vi "查找文件或文件夹.vi"(6 "create file or folder？":bool=TRUE, 8 "error in":errorcluster, 11 "pathIn":path caption="路径") -> (0 "error out":errorcluster, 2 "file or folder exists?":bool caption="文件或文件夹存在？", 3 "pathOut":path)   [LabVIEW 2014]
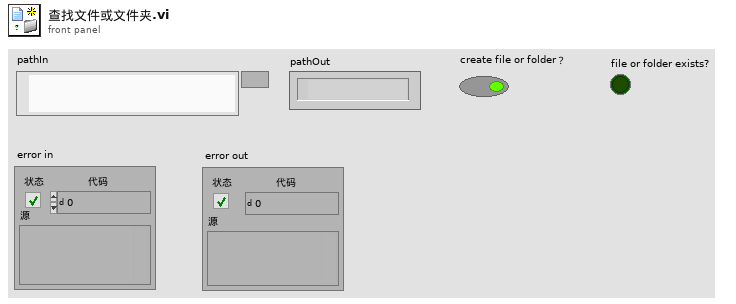
[diagram p1: front panel]
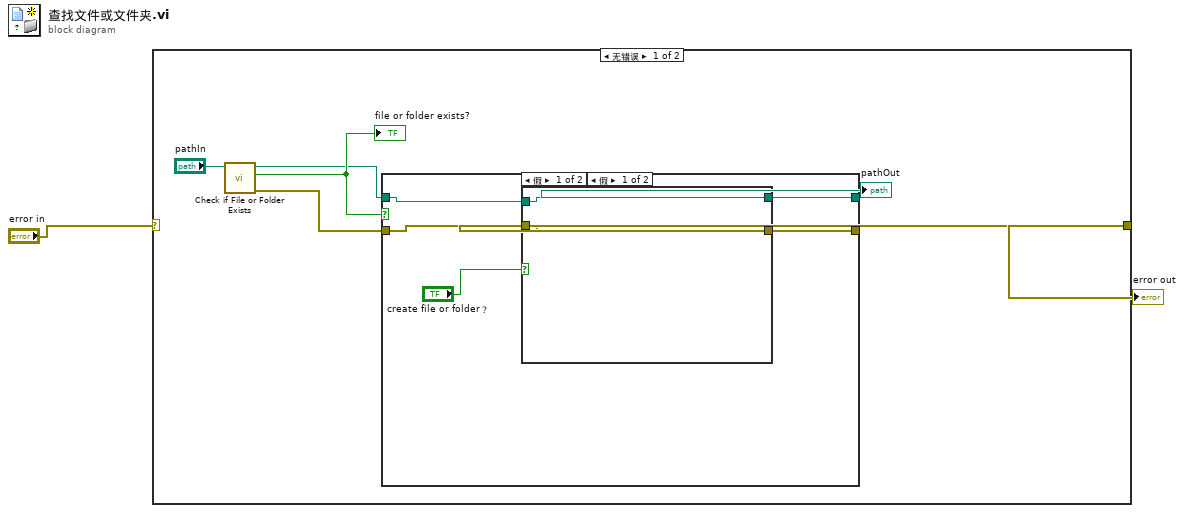
[diagram p0: block diagram]
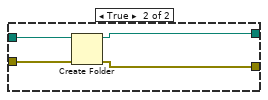
[diagram p2: hidden frame]
diagram:
  n1 = case shown="无错误" "error in" {
    selector: "error in" -> [_ w22]
    tunnel: [w3 w22] -> w1
    frame No Error {
      n2 = call <vilib>:"Check if File or Folder Exists.vi"("path"="pathIn") -> ("error out"=w6:errorcluster, "file or folder exists?"=w8:bool, "dup path"=w7:path)  [unwired: 8 in]
      "file or folder exists?" <- w8
      n3 = case shown="假" w8 {
        tunnel: w7 -> [w12 w21]
        tunnel: w6 -> [w13 w20]
        tunnel: [w11 w21] -> w4
        tunnel: [w10 w20] -> w3
        frame False {
          n4 = case shown="假" "create file or folder？" {
            tunnel: w13 -> [w15 w19]
            tunnel: w12 -> [w14 w18]
            tunnel: [w14 w17] -> w11
            tunnel: [w15 w16] -> w10
            frame False {
            }
            frame True {
              n5 = Create Folder(path (use dialog)=w18, error in=w19) -> (created path=w17:path, error out=w16:errorcluster)  [unwired: 1 in, 1 out]
            }
          }
        }
        frame True {
        }
      }
      "pathOut" <- w4
    }
    frame Error {
    }
  }
  "error out" <- w1
